vi "IOScan_SetRowAndColSizes.vi"(8 "error in":errorcluster, 10 "Configurable Faults in":refnum<vi>, 11 "Choice Ring in":refnum<vi>) -> (0 "error out":errorcluster, 2 "Configurable Faults Out":refnum<vi>, 3 "Choice Ring out":refnum<vi>)   [LabVIEW 2016]
uses:
  <vilib>/Utility/miscctls.llb/LVRowAndColumnTypeDef.ctl
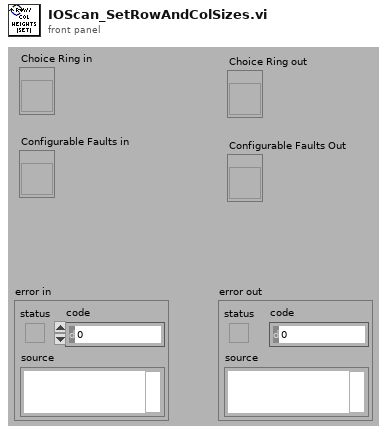
[diagram p1: front panel]
types:
  T1 = typedef "LVRowAndColumnTypeDef.ctl" = cluster{"Row":i32, "Column":i32}
  T2 = typedef "LVBoundsTypeDef.ctl" = cluster{"Width":u32, "Height":u32}
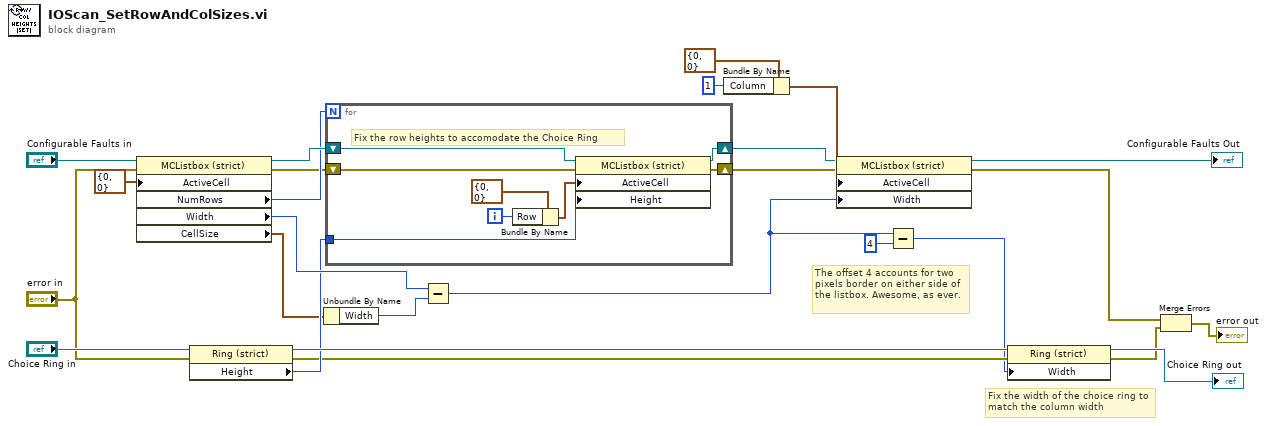
[diagram p0: block diagram]
diagram:
  # "The offset 4 accounts for two pixels border on either side of the listbox. Awesome, as ever."
  # "Fix the width of the choice ring to match the column width"
  n1 = property class="MCListbox (strict)"(reference="Configurable Faults in", error in="error in", "ActiveCell"=T1 {"Row"=0, "Column"=0} ("Active Cell:Active Cell")) -> (reference out=w11:refnum<vi>, error out=w7:errorcluster, "NumRows"=w10:u32, "Width"=w22:u32, "CellSize"=w8:T2)
  n2 = property class="Ring (strict)"(reference="Choice Ring in", error in="error in") -> (reference out=w17:refnum<vi>, error out=w4:errorcluster, "Height"=w12:u32)
  n3 = Unbundle By Name(w8) -> ("Width"=w5:u32)
  n4 = for {
    N: w10 -> [_]
    shift-right: [w28] -> w15
    shift-left: w11 -> [w34]
    shift-right: [w29] -> w16
    shift-left: w7 -> [w27]
    tunnel: w12 -> [w30]
    i -> [w31]
    # "Fix the row heights to accomodate the Choice Ring"
    n5 = Bundle By Name(cluster=T1 {"Row"=0, "Column"=0} ("Active Cell:Active Cell"), "Row"=w31) -> (w32:T1)
    n6 = property class="MCListbox (strict)"(reference=w34, error in=w27, "ActiveCell"=w32, "Height"=w30) -> (reference out=w28:refnum<vi>, error out=w29:errorcluster)
  }
  n7 = Subtract(x=w22, y=w5) -> (x-y=w3:u32)
  n8 = Bundle By Name(cluster=T1 {"Row"=0, "Column"=0} ("Active Cell:Active Cell"), "Column"=1) -> (w20:T1)
  n9 = property class="MCListbox (strict)"(reference=w15, error in=w16, "ActiveCell"=w20, "Width"=w3) -> (reference out=→"Configurable Faults Out":refnum<vi>, error out=w24:errorcluster)
  n10 = Subtract(x=w3, y=u32 4) -> (x-y=w1:u32)
  n11 = property class="Ring (strict)"(reference=w17, error in=w4, "Width"=w1) -> (reference out=→"Choice Ring out":refnum<vi>, error out=w23:errorcluster)
  n12 = Merge Errors(w24, w23) -> (→"error out":errorcluster)
